vi "qHID.vi"(0 "System no.":i32=1 min=1 max=4 step=1, 3 "Invert order?":bool, 5 "error in":errorcluster) -> (14 "Hidden axes":string[](array[string]), 19 "error out":errorcluster)   [LabVIEW 2026]
doc: "Replies which axes are hidden on the controller screen.\n\nC-702: Invert order should be TRUE\nC-848: Invert order should be TRUE\nC-880: Invert order should be TRUE"
uses:
  Communication/Global1.vi
panel:
  # "Replies which axes are hidden on the controller screen."
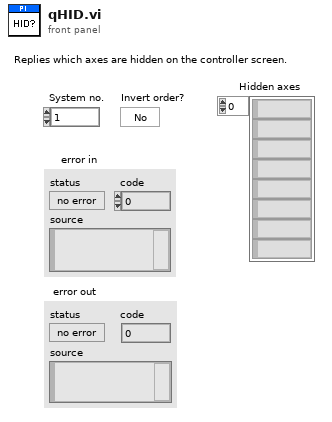
[diagram p1: front panel]
types:
  T1 = typedef "Syntax.ctl" = enum16{"GCS 1.0", "GCS 2.0", "GCS 3.0"}
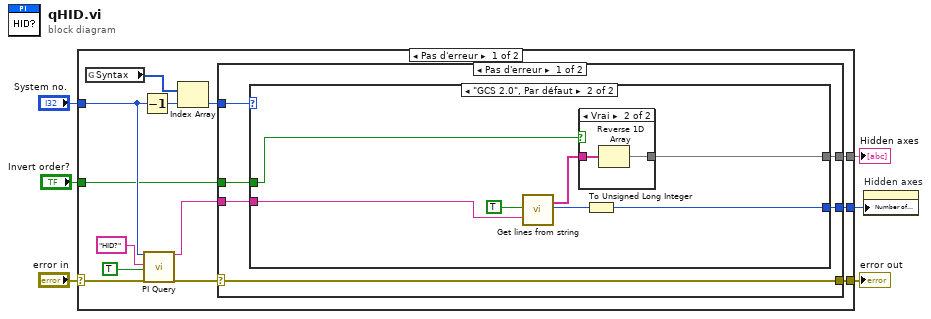
[diagram p0: block diagram]
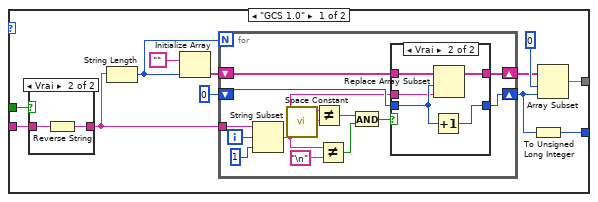
[diagram p2: hidden frame]
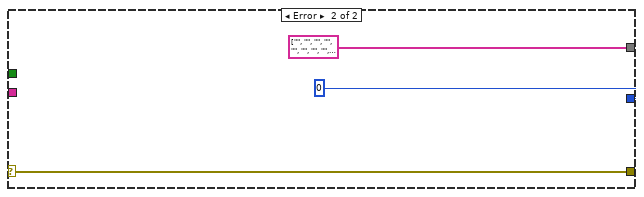
[diagram p6: hidden frame]
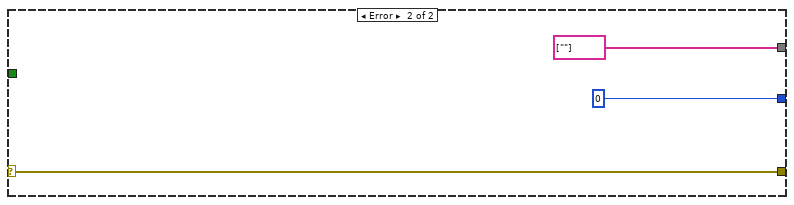
[diagram p7: hidden frame]
diagram:
  n1 = case shown="Pas d'erreur" "error in" {
    selector: "error in" -> [w11 w76]
    tunnel: "System no." -> [w15 _]
    tunnel: [w14 string[] [""] ("Strings")] -> w5
    tunnel: [w13 u32 0 ("Array size out")] -> w4
    tunnel: [w8 w76] -> w3
    tunnel: "Invert order?" -> [w7 _]
    frame No Error {
      n2 = global read "Global1.vi" "Syntax"() -> (w16:T1[])
      n3 = Decrement(x=w15) -> (x-1=w17:i32)
      n4 = call "PI Query.vi"("System no."=w15, "String to send"="HID?", "Attach termination char.?"=TRUE ("Attach Linefeed?"), "error in"=w11) -> ("String read"=w12:string, "error out"=w9:errorcluster)  [unwired: 3 in, 11 out]
      n5 = Index Array(array=w16, index=w17) -> (element=w10:T1)
      n6 = case shown="Pas d'erreur" w9 {
        selector: w9 -> [w20 w71]
        tunnel: w12 -> [w22 _]
        tunnel: [w25 u32 0] -> w13
        tunnel: [w24 string[] ["", "", "", "", "", "", "", "", "", "", "", "", "", "", "", "", "", "", "", "", "", "", "", "", "", "", ""] ("Conn. Axes 2")] -> w14
        tunnel: w7 -> [w23 _]
        tunnel: w10 -> [w21 _]
        tunnel: [w20 w71] -> w8
        frame No Error {
          n7 = case shown="\"GCS 2.0\", Par défaut" w21 {
            tunnel: [w26 w61] -> w25
            tunnel: [w30 w63] -> w24
            tunnel: w23 -> [w28 w62]
            tunnel: w22 -> [w27 w65]
            frame "GCS 1.0" {
              n8 = case shown="Vrai" w28 {
                tunnel: w27 -> [w38 w40]
                tunnel: [w38 w39] -> w29
                frame False {
                }
                frame True {
                  n9 = Reverse String(1:w40) -> (0:w39:string)
                }
              }
              n10 = String Length(string=w29) -> (length=w36:i32)
              n11 = Initialize Array("" ("Element Data"), w36) -> (w34:string[])
              n12 = for {
                N: w36 -> [_]
                tunnel: w29 -> [w53]
                shift-right: [w46] -> w31
                shift-left: w34 -> [w47]
                shift-right: [w49] -> w32
                shift-left: 0 -> [w48]
                i -> [w51]
                n13 = String Subset(string=w53, offset (0)=w51, length (rest)=1 ("length")) -> (substring=w45:string)
                n14 = call <vilib>:"Space Constant.vi"() -> ("String"=w50:string)
                n15 = Not Equal?(x=w45, y=w50) -> (x != y?=w43:bool)
                n16 = Not Equal?(x=w45, y="\n") -> (x != y?=w42:bool)
                n17 = And(x=w43, y=w42) -> (x .and. y?=w41:bool)
                n18 = case shown="Vrai" w41 {
                  tunnel: [w55 w60] -> w49
                  tunnel: w48 -> [w55 w58]
                  tunnel: w47 -> [w54 w59]
                  tunnel: w45 -> [_ w57]
                  tunnel: [w54 w56] -> w46
                  frame False {
                  }
                  frame True {
                    n19 = Increment(x=w58) -> (x+1=w60:i32)
                    n20 = Replace Array Subset(array=w59, new element=w57, index=w58) -> (w56:string[])
                  }
                }
              }
              n21 = To Unsigned Long Integer(number=w32) -> (unsigned 32bit integer=w26:u32)
              n22 = Array Subset(array=w31, index=0 ("Array Index"), length=w32) -> (w30:string[])
            }
            frame "GCS 2.0", Default {
              n23 = call "Get lines from string.vi"("Cut spaces?"=TRUE, "Input string"=w65) -> ("Strings"=w66:string[], "Array size out"=w64:i32)  [unwired: 1 in, 15 out]
              n24 = case shown="Vrai" w62 {
                tunnel: w66 -> [w68 w70]
                tunnel: [w68 w69] -> w63
                frame False {
                }
                frame True {
                  n25 = Reverse 1D Array(array=w70) -> (reversed array=w69:string[])
                }
              }
              n26 = To Unsigned Long Integer(number=w64) -> (unsigned 32bit integer=w61:u32)
            }
          }
        }
        frame Error {
        }
      }
    }
    frame Error {
    }
  }
  "error out" <- w3
  "Hidden axes" <- w5
  n27 = property on="Hidden axes" class="Tabl (strict)"("Number of Rows"=w4) -> ()  [unwired: 2 in, 2 out]
